vi "3C Helper - Wrap around.vi"(9 "Range allowed":dbl=10.0, 10 "Min allowed":dbl, 11 "Position in":dbl) -> (3 "Wrapped Position out":dbl)   [LabVIEW 2011]
doc: "Takes an input and moves it into a given range, defined by a minimum and a range size. Moves the input by up to the range size given. Note this means that if the input is outside the range by more than the size of the range, it will not successfully be pulled into the range."
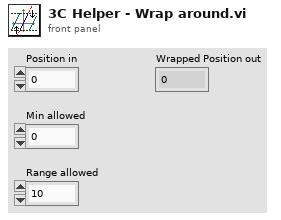
[diagram p1: front panel]
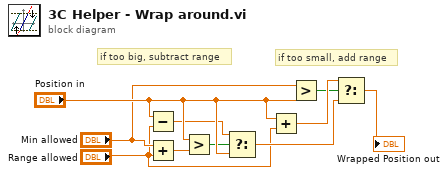
[diagram p0: block diagram]
diagram:
  # "if too small, add range"
  # "if too big, subtract range"
  n1 = Subtract(x="Position in", y="Range allowed") -> (x-y=w6:dbl)
  n2 = Add(x="Min allowed", y="Range allowed") -> (x+y=w5:dbl)
  n3 = Greater?(x="Position in", y=w5) -> (0:w2:bool)
  n4 = Select(t=w6, s=w2, f="Position in") -> (s? t:f=w7:dbl)
  n5 = Add(x="Position in", y="Range allowed") -> (x+y=w9:dbl)
  n6 = Greater?(x="Min allowed", y="Position in") -> (0:w4:bool)
  n7 = Select(t=w9, s=w4, f=w7) -> (s? t:f=→"Wrapped Position out":dbl)
